vi "calculate_ampl_with_attenuator.vi"(7 "Attenuator(dB)":T10, 8 "error in":errorcluster, 9 "Amplitude_in":dbl, 10 "frequency":dbl, 11 "app_data in in":T1) -> (0 "error out":errorcluster, 2 "Amplitude_out":dbl, 3 "app_data out":T1)   [LabVIEW 2017]
uses:
  controls/app_data.ctl
  controls/instruments.ctl
  Unicorn Labview Library/Control/unicorn_Param.ctl
  Unicorn Labview Library/Control/unicorn_conn.ctl
  Unicorn Labview Library/Control/unicorn_JSON.ctl
  Unicorn Labview Library/Control/unicorn_ParamInt.ctl
  Unicorn Labview Library/Control/unicorn_Telemetry.ctl
  Unicorn Labview Library/Control/unicorn_Table.ctl
  Unicorn Labview Library/Control/unicorn_ParamFloat.ctl
  controls/attenuator_dB.ctl
  Unicorn Labview Library/Unicorn Library.lvlib
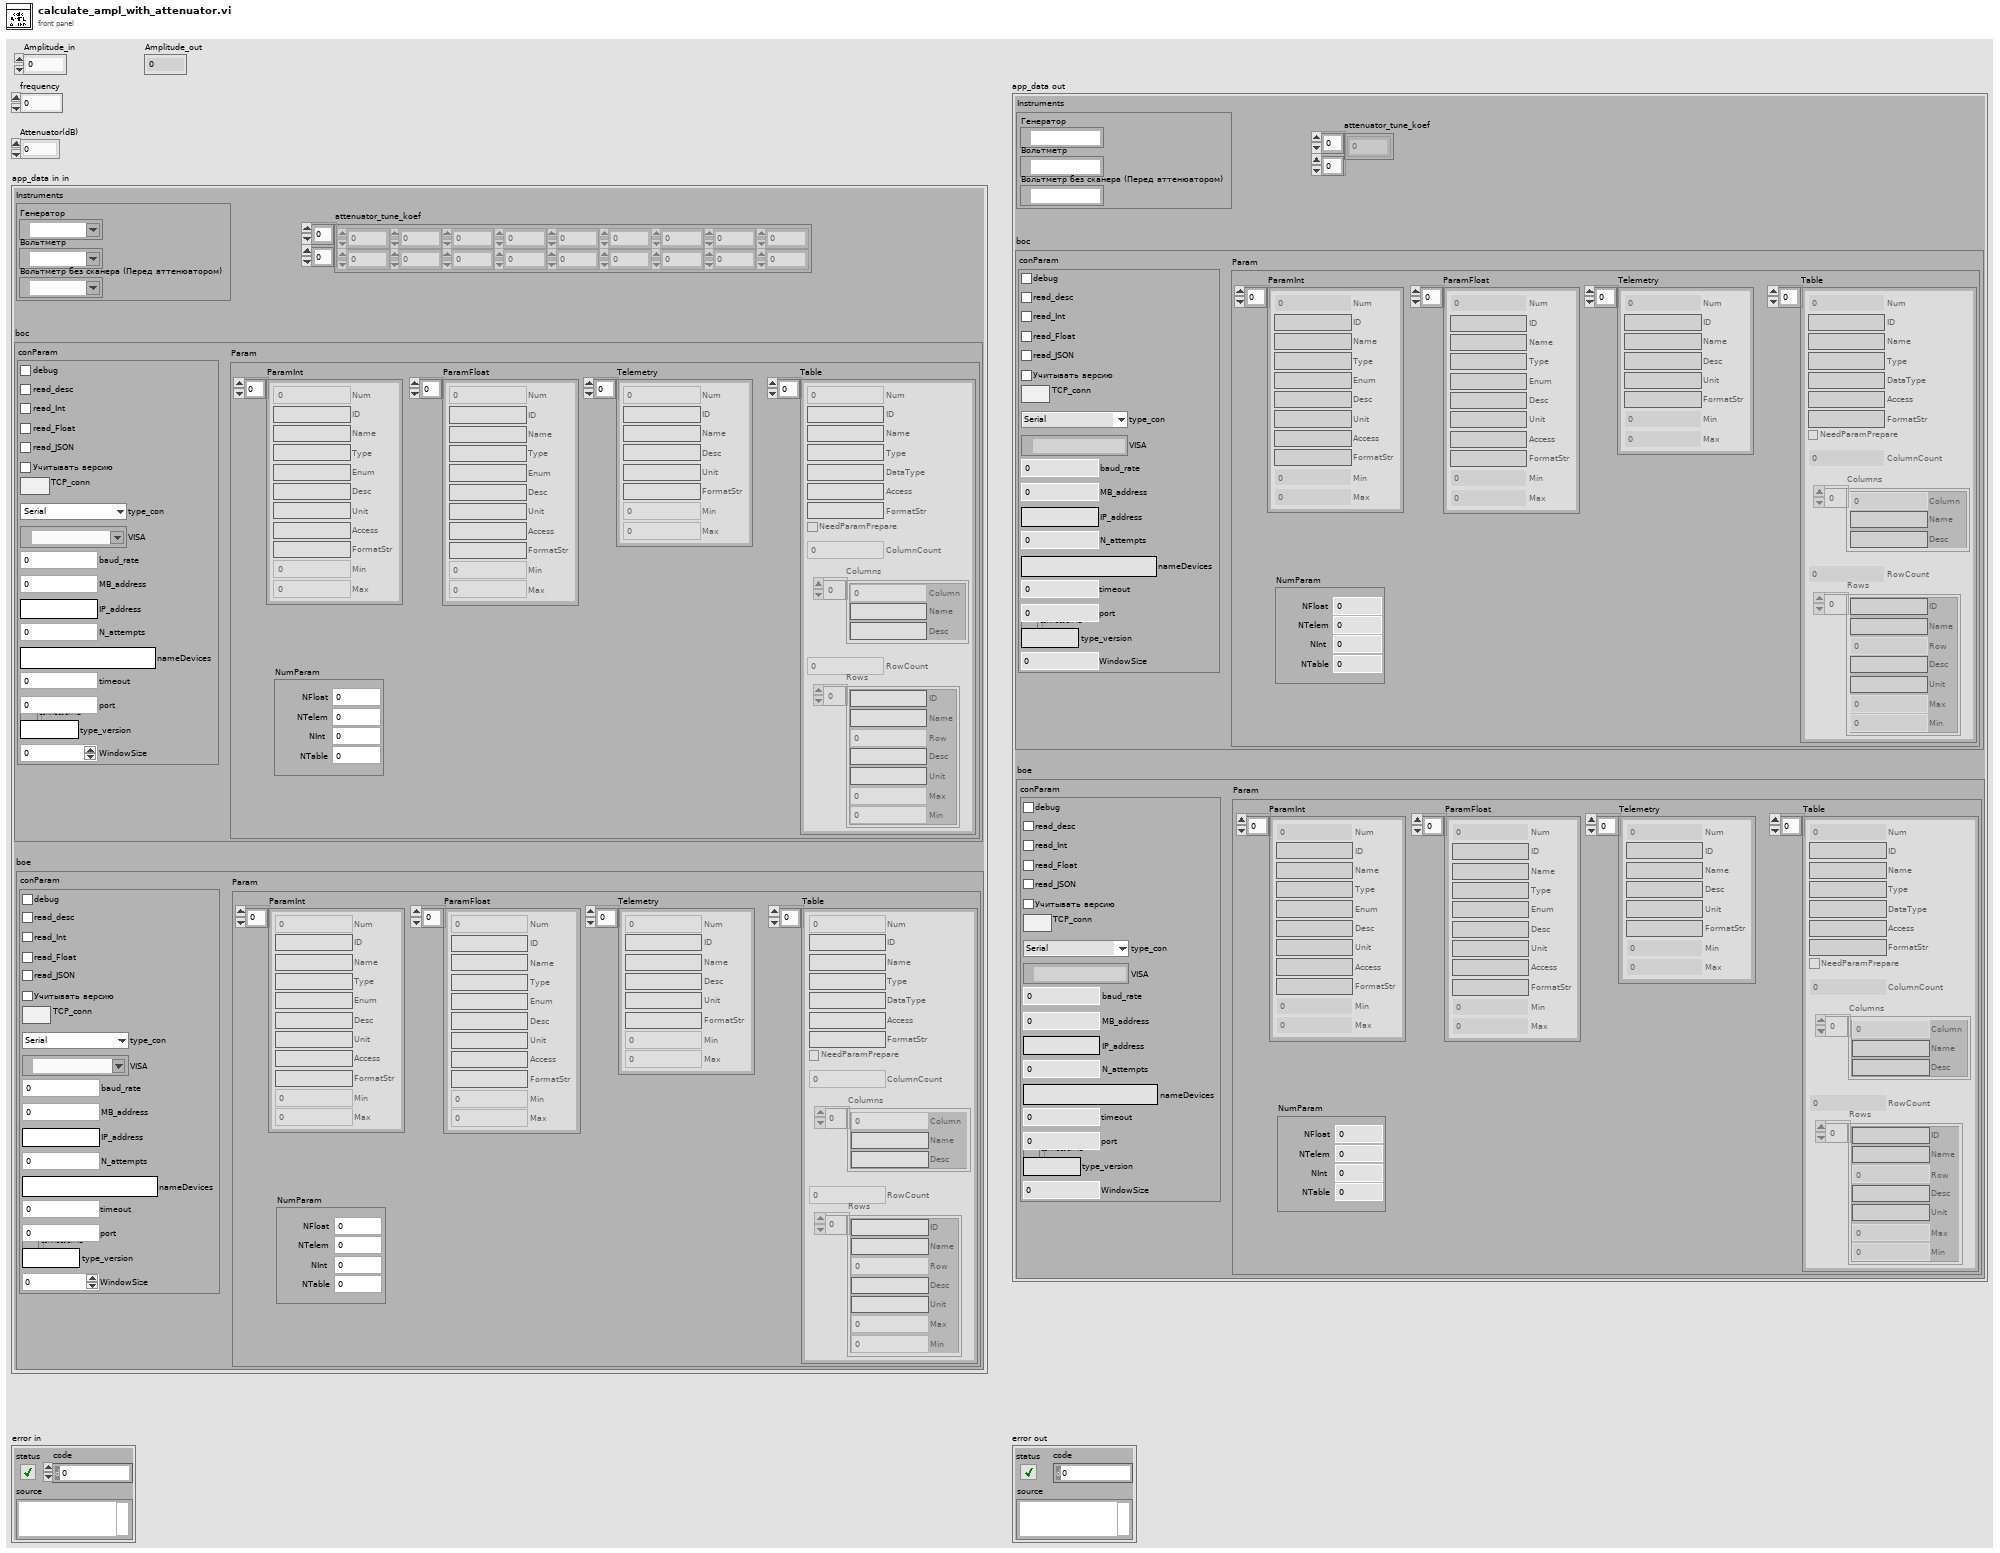
[diagram p1: front panel]
types:
  T1 = typedef "app_data.ctl" = cluster{"Instruments":T2, "boc":T3, "boe":T3, "attenuator_tune_koef":dbl[][]}
  T2 = typedef "instruments.ctl" = cluster{"generator":refnum<visa-resource-name>, "voltment_with_scaner":refnum<visa-resource-name>, "voltment_without_scaner":refnum<visa-resource-name>}
  T3 = typedef "Unicorn Library.lvlib/unicorn_Param.ctl" = cluster{"conParam":T4, "Param":T5}
  T4 = typedef "Unicorn Library.lvlib/unicorn_conn.ctl" = cluster{"ReadIntParam":bool, "ReadDescrParam":bool, "ReadFloatParam":bool, "debug":bool, "ReadJSON":bool, "IP_address":string, "N_attempts":i32, "type_con":enum16{"Serial", "TCP"}, "MB_address":i32, "VISA":refnum<visa-resource-name>, "connection ID":refnum<k5>, "nameDevices":string, "timeout":i32, "port":u16, "type_version":string, "baud_rate":u32, "VersionControl":bool, "TCP_conn":bool, "WindowSize":i32}
  T5 = typedef "Unicorn Library.lvlib/unicorn_JSON.ctl" = cluster{"NumParam":cluster{"NTelem":i32, "NInt":i32, "NFloat":i32, "NTable":i32}, "ParamInt":T6, "Telemetry":T7, "Table":T8, "ParamFloat":T9}
  T6 = typedef "Unicorn Library.lvlib/unicorn_ParamInt.ctl" = cluster{"ID":string, "Num":i32, "Name":string, "Type":string, "Enum":string, "Desc":string, "Unit":string, "Access":string, "FormatStr":string, "Min":i32, "Max":i32}[]
  T7 = typedef "Unicorn Library.lvlib/unicorn_Telemetry.ctl" = cluster{"ID":string, "Num":i32, "Name":string, "Desc":string, "Unit":string, "FormatStr":string, "Min":i32, "Max":i32}[]
  T8 = typedef "Unicorn Library.lvlib/unicorn_Table.ctl" = cluster{"Num":i32, "Access":string, "ColumnCount":i32, "NeedParamPrepare":bool, "Columns":cluster{"Column":i32, "Desc":string, "Name":string}[], "DataType":string, "FormatStr":string, "ID":string, "Name":string, "RowCount":i32, "Rows":cluster{"Desc":string, "ID":string, "Max":i32, "Min":i32, "Name":string, "Row":i32, "Unit":string}[], "Type":string}[]
  T9 = typedef "Unicorn Library.lvlib/unicorn_ParamFloat.ctl" = cluster{"ID":string, "Num":i32, "Name":string, "Type":string, "Enum":string, "Desc":string, "Unit":string, "Access":string, "FormatStr":string, "Min":i32, "Max":i32}[]
  T10 = typedef "attenuator_dB.ctl" = enum16{"0", "20", "40", "60"}
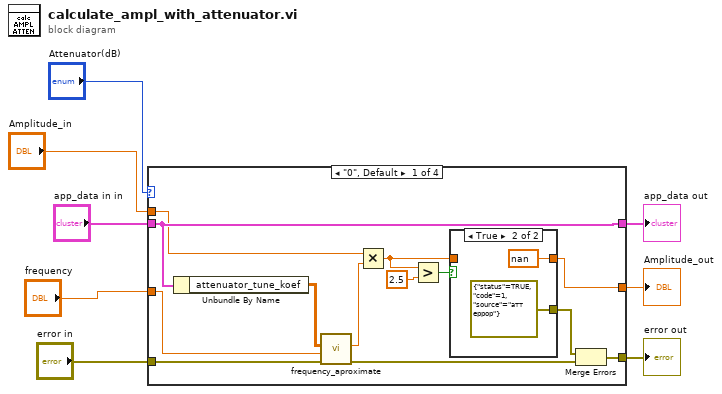
[diagram p0: block diagram]
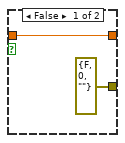
[diagram p2: hidden frame]
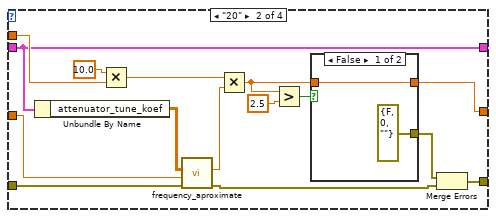
[diagram p3: hidden frame]
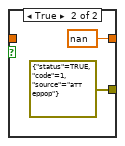
[diagram p4: hidden frame]
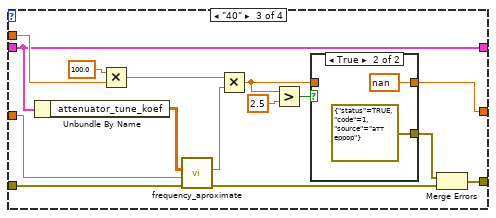
[diagram p5: hidden frame]
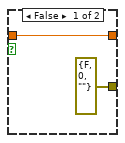
[diagram p6: hidden frame]
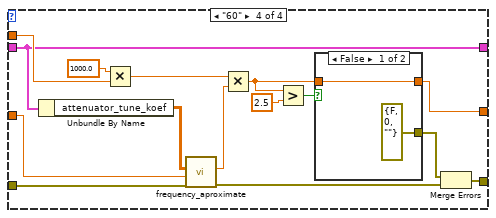
[diagram p7: hidden frame]
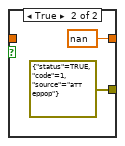
[diagram p8: hidden frame]
diagram:
  n1 = case shown="\"0\", Default" "Attenuator(dB)" {
    tunnel: "app_data in in" -> [w14 w33 w47 w68]
    tunnel: "frequency" -> [w13 w39 w49 w65]
    tunnel: "error in" -> [w12 w38 w48 w64]
    tunnel: [w10 w27 w45 w66] -> w4
    tunnel: "Amplitude_in" -> [w9 w34 w50 w69]
    tunnel: [w14 w33 w47 w68] -> w7
    tunnel: [w11 w30 w46 w67] -> w8
    frame "0", Default {
      n2 = Unbundle By Name(w14) -> ("attenuator_tune_koef"=w21:dbl[][])
      n3 = call "frequency_aproximate.vi"("error_in"=w12, "freq"=w13, "Array"=w21) -> ("error_out"=w16:errorcluster, "koef"=w20:dbl)  [unwired: 7 in]
      n4 = Multiply(x=w9, y=w20) -> (x*y=w15:dbl)
      n5 = Greater?(x=w15, y=2.5) -> (0:w18:bool)
      n6 = case shown="True" w18 {
        tunnel: [w23 nan ("Amplitude (1.0 Vpp)")] -> w11
        tunnel: [errorcluster {"status"=FALSE, "code"=0, "source"=""} ("error constant") errorcluster {"status"=TRUE, "code"=1, "source"="атт еррор"} ("error constant")] -> w17
        tunnel: w15 -> [w23 _]
        frame False {
        }
        frame True {
        }
      }
      n7 = Merge Errors(w17, w16) -> (w10:errorcluster)
    }
    frame "20" {
      n8 = Unbundle By Name(w33) -> ("attenuator_tune_koef"=w40:dbl[][])
      n9 = Multiply(x=10.0, y=w34) -> (x*y=w37:dbl)
      n10 = call "frequency_aproximate.vi"("error_in"=w38, "freq"=w39, "Array"=w40) -> ("error_out"=w28:errorcluster, "koef"=w35:dbl)  [unwired: 7 in]
      n11 = Multiply(x=w37, y=w35) -> (x*y=w26:dbl)
      n12 = Greater?(x=w26, y=2.5) -> (0:w31:bool)
      n13 = case shown="False" w31 {
        tunnel: [w42 nan ("Amplitude (1.0 Vpp)")] -> w30
        tunnel: [errorcluster {"status"=FALSE, "code"=0, "source"=""} ("error constant") errorcluster {"status"=TRUE, "code"=1, "source"="атт еррор"} ("error constant")] -> w29
        tunnel: w26 -> [w42 _]
        frame False {
        }
        frame True {
        }
      }
      n14 = Merge Errors(w29, w28) -> (w27:errorcluster)
    }
    frame "40" {
      n15 = Unbundle By Name(w47) -> ("attenuator_tune_koef"=w59:dbl[][])
      n16 = Multiply(x=100.0, y=w50) -> (x*y=w58:dbl)
      n17 = call "frequency_aproximate.vi"("error_in"=w48, "freq"=w49, "Array"=w59) -> ("error_out"=w52:errorcluster, "koef"=w56:dbl)  [unwired: 7 in]
      n18 = Multiply(x=w58, y=w56) -> (x*y=w51:dbl)
      n19 = Greater?(x=w51, y=2.5) -> (0:w54:bool)
      n20 = case shown="True" w54 {
        tunnel: [w61 nan ("Amplitude (1.0 Vpp)")] -> w46
        tunnel: [errorcluster {"status"=FALSE, "code"=0, "source"=""} ("error constant") errorcluster {"status"=TRUE, "code"=1, "source"="атт еррор"} ("error constant")] -> w53
        tunnel: w51 -> [w61 _]
        frame False {
        }
        frame True {
        }
      }
      n21 = Merge Errors(w53, w52) -> (w45:errorcluster)
    }
    frame "60" {
      n22 = Unbundle By Name(w68) -> ("attenuator_tune_koef"=w78:dbl[][])
      n23 = Multiply(x=1000.0, y=w69) -> (x*y=w77:dbl)
      n24 = call "frequency_aproximate.vi"("error_in"=w64, "freq"=w65, "Array"=w78) -> ("error_out"=w71:errorcluster, "koef"=w75:dbl)  [unwired: 7 in]
      n25 = Multiply(x=w77, y=w75) -> (x*y=w70:dbl)
      n26 = Greater?(x=w70, y=2.5) -> (0:w73:bool)
      n27 = case shown="False" w73 {
        tunnel: [w80 nan ("Amplitude (1.0 Vpp)")] -> w67
        tunnel: [errorcluster {"status"=FALSE, "code"=0, "source"=""} ("error constant") errorcluster {"status"=TRUE, "code"=1, "source"="атт еррор"} ("error constant")] -> w72
        tunnel: w70 -> [w80 _]
        frame False {
        }
        frame True {
        }
      }
      n28 = Merge Errors(w72, w71) -> (w66:errorcluster)
    }
  }
  "Amplitude_out" <- w8
  "app_data out" <- w7
  "error out" <- w4
